vi "Get Sub Panel.vi"(10 "index":i32, 11 "banner gui refs":T1[](array[typedef])) -> (3 "selected vi":refnum<vi>)   [LabVIEW 2020]
uses:
  GUI References.ctl
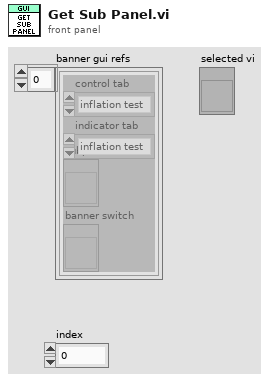
[diagram p1: front panel]
types:
  T1 = typedef "GUI References.ctl" = cluster{"control tab":enum32{"inflation test", "force calibration", "camera calibration", "test equipment"}, "indicator tab":enum32{"inflation test", "force calibration", "camera calibration", "test equipment"}, "subpanel vi":refnum<vi>, "banner switch":refnum<vi>}
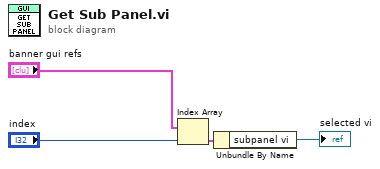
[diagram p0: block diagram]
diagram:
  n1 = Index Array(array="banner gui refs", index="index") -> (element=w3:T1)
  n2 = Unbundle By Name(w3) -> ("subpanel vi"=→"selected vi":refnum<vi>)
